vi "PVCamPropertyChangedEventCallbackForBufferIndexDroppedFrame.vi"(4 "User Parameter":cluster{refnum<vi>, refnum<vi>, refnum<vi>}, 5 "Event Data":cluster{"sender":refnum<k24>, "e":refnum<k24>}, 6 "Control Ref":refnum<k24>, 7 "Event Common Data":T1) -> ()   [LabVIEW 2019]
uses:
  Dependencies/PVCamNET.dll
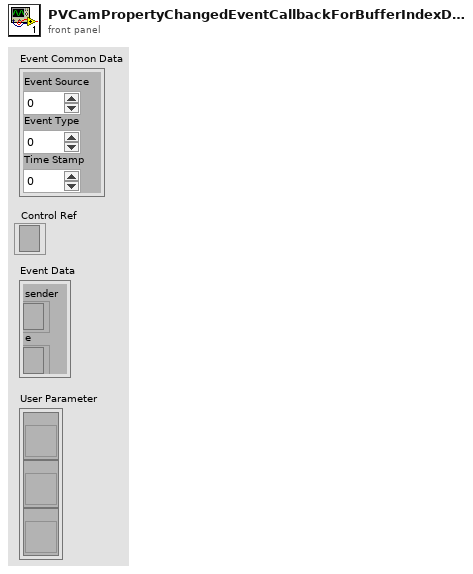
[diagram p1: front panel]
types:
  T1 = cluster{"Event Source":i32, "Event Type":u32, "Time Stamp":u32}
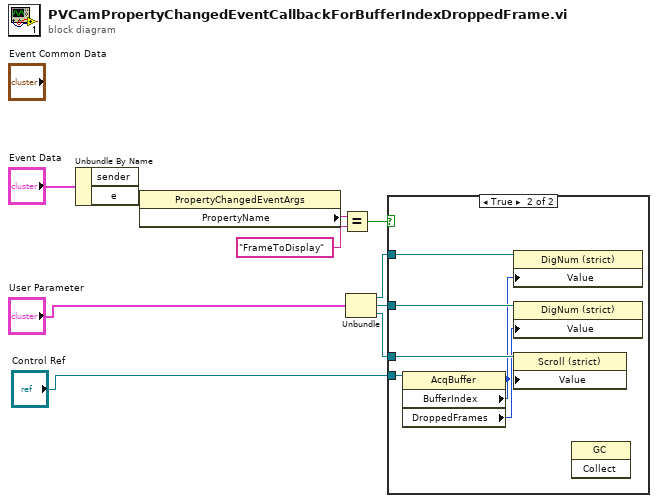
[diagram p0: block diagram]
diagram:
  n1 = Unbundle By Name("Event Data") -> ("e"=w10:refnum<k24>)  [unwired: 1 out]
  n2 = property class="PropertyChangedEventArgs"(reference=w10) -> ("PropertyName"=w9:string)  [unwired: 1 in, 2 out]
  n3 = Equal?(x=w9, y="FrameToDisplay") -> (x = y?=w7:bool)
  n4 = Unbundle("User Parameter") -> (w4:refnum<vi>, w3:refnum<vi>, w2:refnum<vi>)
  n5 = case shown="True" w7 {
    tunnel: w4 -> [_ w16]
    tunnel: "Control Ref" -> [_ w15]
    tunnel: w3 -> [_ w14]
    tunnel: w2 -> [_ w13]
    frame False {
    }
    frame True {
      n6 = property class="AcqBuffer"(reference=w15) -> ("BufferIndex"=w11:i32, "DroppedFrames"=w12:i32)  [unwired: 1 in, 2 out]
      n7 = property class="DigNum (strict)"(reference=w16, "Value"=w11) -> ()  [unwired: 1 in, 2 out]
      n8 = property class="DigNum (strict)"(reference=w14, "Value"=w12) -> ()  [unwired: 1 in, 2 out]
      n9 = property class="Scroll (strict)"(reference=w13, "Value"=w11) -> ()  [unwired: 1 in, 2 out]
      n10 = invoke class="GC" method="Collect"() -> ()  [unwired: 3 in, 3 out]
    }
  }
